vi "Draw Badges.vi"(8 "error in (no error)":errorcluster, 10 "picture in":picture, 11 "FSM in":refnum<class "FSM.Node.lvclass">) -> (0 "error out":errorcluster, 2 "picture out":picture, 3 "FSM out":refnum<class "FSM.Node.lvclass">)   [LabVIEW 2015, in "FSM.Node.lvclass"]
uses:
  FSM.Node.lvclass
  FSM.Node.lvclass/FSM.Node.ctl
  <vilib>/picture/picture.llb/Draw True-Color Pixmap.vi
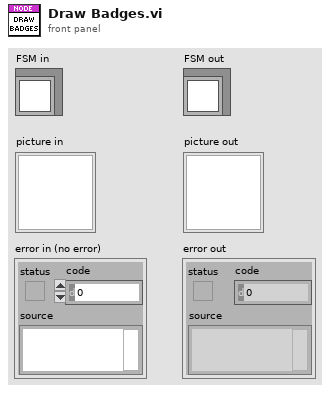
[diagram p1: front panel]
types:
  T1 = typedef "FSM.Node.lvclass/Badge.ctl" = enum16{"Audio", "Visual"}
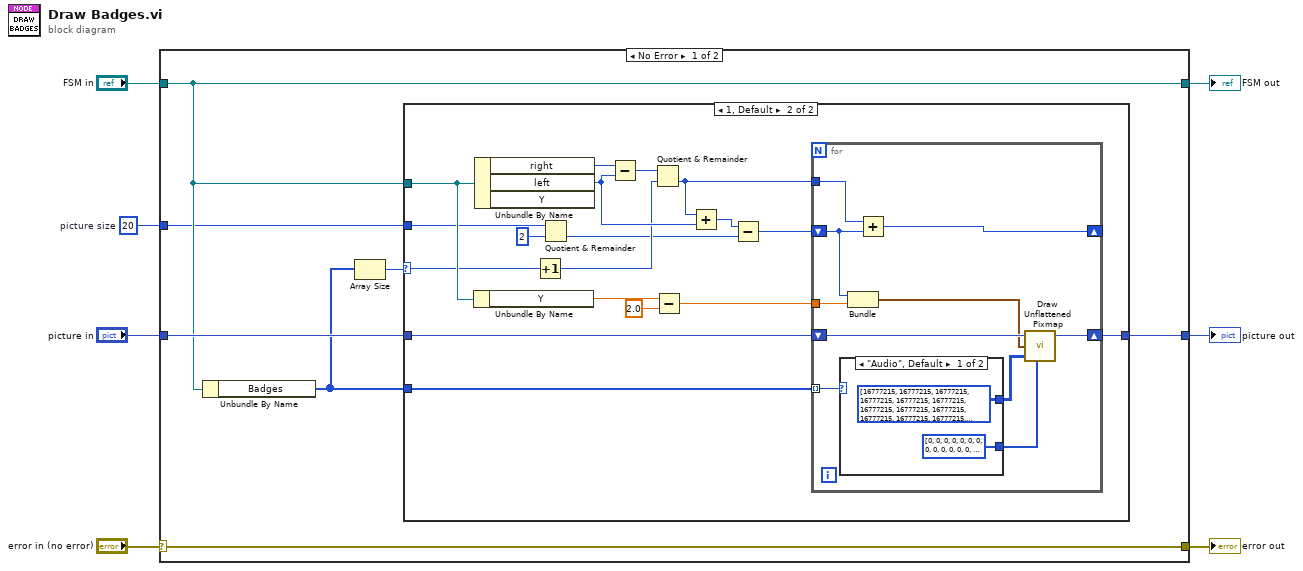
[diagram p0: block diagram]
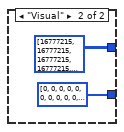
[diagram p3: hidden frame]
diagram:
  w1 = 20  # picture size
  n1 = case shown="No Error" "error in (no error)" {
    selector: "error in (no error)" -> [w14 w50]
    tunnel: [w14 w50] -> w6
    tunnel: [w11 w49] -> w4
    tunnel: "FSM in" -> [w11 w49]
    tunnel: "picture in" -> [w13 w48]
    tunnel: [w12 w48] -> w2
    tunnel: w1 -> [w9 _]
    frame No Error {
      n2 = Unbundle By Name(w11) -> ("Badges"=w8:T1[])
      n3 = Array Size(array=w8) -> (size(s)=w10:i32)
      n4 = case shown="1, Default" w10 {
        selector: w10 -> [_ w24]
        tunnel: w13 -> [w15 w31]
        tunnel: [w15 w30] -> w12
        tunnel: w11 -> [_ w27]
        tunnel: w9 -> [_ w23]
        tunnel: w8 -> [_ w20]
        frame 0 {
        }
        frame 1, Default {
          n5 = Unbundle By Name(w27) -> ("Y"=w26:dbl)
          n6 = Unbundle By Name(w27) -> ("right"=w33:i16, "left"=w29:i16)  [unwired: 1 out]
          n7 = Increment(x=w24) -> (x+1=w25:i32)
          n8 = Quotient & Remainder(x=w23, y=2) -> (floor(x/y)=w21:i32)  [unwired: 1 out]
          n9 = Subtract(x=w33, y=w29) -> (x-y=w32:i16)
          n10 = Quotient & Remainder(x=w32, y=w25) -> (floor(x/y)=w16:i32)  [unwired: 1 out]
          n11 = Subtract(x=w26, y=2.0) -> (x-y=w18:dbl)
          n12 = Add(x=w16, y=w29) -> (x+y=w17:i32)
          n13 = Subtract(x=w17, y=w21) -> (x-y=w19:i32)
          n14 = for {
            shift-right: [w42] -> w30
            shift-left: w31 -> [w43]
            tunnel: w20 -> [w34] mode=indexing
            tunnel: w18 -> [w39]
            tunnel: w16 -> [w37]
            shift-right: [w35] -> _
            shift-left: w19 -> [w36]
            n15 = case shown="\"Audio\", Default" w34 {
              tunnel: [u32[][] [[16777215, 16777215, 16777215, 16777215, 16777215, 16777215, 16777215, 16777215, 16777215, 16777215, 16777215, 16777215, 16777215, 16777215, 16777215, 16777215, 16777215, 16777215, 16777215, 16777215], [16777215, 16777215, 16777215, 16777215, 16777215, 16777215, 16777215, 16777215, 16777215, 16777215, 16777215, 16777215, 16777215, 16777215, 16777215, 16777215, 16777215, 16777215, 16777215, 16777215], [16777215, 16777215, 16777215, 16777215, 16777215, 16777215, 16777215, 16777215, 16777215, 16777215, 16777215, 16777215, 16777215, 16777215, 16777215, 16777215, 16777215, 16777215, 16777215, 16777215], [16777215, 16777215, 16777215, 16777215, 16777215, 16777215, 16777215, 16777215, 16777215, 16777215, 16777215, 16777215, 16777215, 16777215, 16777215, 16777215, 16777215, 16777215, 16777215, 16777215], [16777215, 16777215, 16777215, 5994709, 5994709, 5994709, 5994709, 5994709, 5863381, 5797332, 10464994, 14804723, 8228815, 12634601, 15922427, 16382718, 16514046, 16777215, 16777215, 16777215], [16777215, 16777215, 16777215, 4746200, 4746200, 4746200, 4746200, 4746200, 4811992, 4680665, 2772939, 4678084, 7439820, 14673139, 16054012, 16382717, 16514046, 16777215, 16777215, 16777215], [16777215, 16777215, 16777215, 1653428, 1653428, 1653428, 1653428, 1653428, 1653428, 1653684, 601519, 3232, 861346, 8229582, 16054012, 16711423, 16448254, 16777215, 16777215, 16777215], [16777215, 16777215, 16777215, 1192870, 1192870, 1192870, 1192870, 1192870, 929957, 1981867, 9280981, 4679099, 4502, 1425, 8491471, 16777215, 16777215, 16777215, 16777215, 16777215], [16777215, 16777215, 16777215, 1192866, 1192866, 1192866, 1192866, 1192866, 929952, 1653157, 9017810, 11911651, 9149652, 5782, 467610, 12897513, 16579839, 16777215, 16777215, 16777215], [16777215, 16777215, 16777215, 7319, 7320, 73112, 1192610, 1324451, 1258659, 798368, 535199, 8360655, 16777215, 11056862, 8599, 7638475, 15067894, 16777215, 16777215, 16777215], [16777215, 16777215, 16777215, 9609942, 9544149, 9084115, 1391267, 1062305, 1522339, 1522596, 8343, 5270459, 16579583, 16777215, 10005468, 3432123, 6061769, 16777215, 16777215, 16777215], [16777215, 16777215, 16777215, 16514046, 16185340, 16645375, 8492753, 538274, 998563, 1458597, 1064099, 801186, 10333915, 16777215, 14409973, 4614597, 3102654, 16777215, 16777215, 16777215], [16777215, 16777215, 16777215, 14936054, 14409970, 15133430, 12765932, 6455244, 343472, 671921, 1328819, 11944, 6521292, 12371434, 10859490, 10727905, 10727905, 16777215, 16777215, 16777215], [16777215, 16777215, 16777215, 14936054, 14475506, 14936053, 11451365, 10135518, 5798350, 608195, 805573, 13245, 10598888, 16777215, 16382461, 16645374, 16645374, 16777215, 16777215, 16777215], [16777215, 16777215, 16777215, 14936054, 14541555, 15527928, 11845863, 9413084, 8885715, 2777815, 1070811, 807384, 4553186, 15396859, 16776957, 16053755, 16053755, 16777215, 16777215, 16777215], [16777215, 16777215, 16777215, 15922427, 14804469, 10136288, 7835351, 6125258, 4152766, 2185940, 1924315, 2318298, 16851, 11913200, 16777214, 16053755, 16053755, 16777215, 16777215, 16777215], [16777215, 16777215, 16777215, 13883631, 10201050, 4743097, 3427498, 1983148, 1396684, 1726162, 1922510, 1856974, 1396940, 3368659, 15922684, 16447996, 15987963, 16777215, 16777215, 16777215], [16777215, 16777215, 16777215, 8491983, 6058425, 2637975, 2377636, 1858254, 1534962, 2778330, 3236046, 3105233, 2908112, 2776527, 11583466, 16645373, 16645373, 16777215, 16777215, 16777215], [16777215, 16777215, 16777215, 9215184, 5205946, 871351, 1993696, 1602041, 2189800, 10597090, 12897000, 12108775, 12174567, 11516900, 11517671, 16448253, 16711166, 16777215, 16777215, 16777215], [16777215, 16777215, 16777215, 12239585, 9808091, 2845659, 1730281, 4421857, 11845605, 16644342, 16381688, 16184567, 16184567, 16184567, 16184568, 16053755, 16053755, 16777215, 16777215, 16777215]] ("24-bit pixmap") u32[][] [[16777215, 16777215, 16777215, 16777215, 16777215, 16777215, 16777215, 16777215, 16777215, 16777215, 16777215, 16777215, 16777215, 16777215, 16777215, 16777215, 16777215, 16777215, 16777215, 16777215], [16777215, 16777215, 16777215, 16777215, 16777215, 16777215, 16777215, 16777215, 16777215, 16777215, 16777215, 16777215, 16777215, 16777215, 16777215, 16777215, 16777215, 16777215, 16777215, 16777215], [16777215, 16777215, 16777215, 16777215, 16777215, 16777215, 16777215, 16777215, 16777215, 16777215, 16777215, 16777215, 16777215, 16777215, 16777215, 16777215, 16777215, 16777215, 16777215, 16777215], [16777215, 16777215, 16777215, 16777215, 16777215, 16777215, 16777215, 16777215, 16777215, 16777215, 16777215, 16777215, 16777215, 16777215, 16777215, 16777215, 16777215, 16777215, 16777215, 16777215], [16777215, 16777215, 16777215, 16579059, 16117212, 15853272, 15852758, 15123848, 14858328, 14858055, 14857795, 14792277, 14992264, 15919065, 15787734, 16116440, 16447215, 16777215, 16777215, 16777215], [16777215, 16777215, 16777215, 16711422, 16315629, 15190938, 15055174, 15914307, 16311883, 16378705, 16443732, 16112968, 15516218, 14790467, 15190680, 16249322, 16579579, 16777215, 16777215, 16777215], [16777215, 16777215, 16777215, 16579322, 15719872, 14856244, 16245061, 16776291, 16776574, 16776612, 16776890, 16710288, 16445278, 15979070, 14855985, 15719354, 16447478, 16777215, 16777215, 16777215], [16777215, 16777215, 16777215, 15917516, 15122299, 15449901, 16642913, 16776876, 16777199, 16777215, 16777215, 16777209, 16710830, 16511073, 15582766, 15122804, 15719873, 16777215, 16777215, 16777215], [16777215, 16777215, 16777215, 15917517, 15188349, 15449899, 16511344, 16776931, 16777215, 16777215, 16777215, 16777215, 16777204, 16643466, 15649582, 15254386, 15719357, 16777215, 16777215, 16777215], [16777215, 16777215, 16777215, 16380911, 15455145, 15054382, 16246105, 16776136, 16777215, 16777215, 16777215, 16777215, 16777205, 16576902, 15384363, 15322262, 16116449, 16777215, 16777215, 16777215], [16777215, 16777215, 16777215, 16711679, 16381683, 14989919, 15715127, 16511344, 16776385, 16777201, 16777210, 16777198, 16776107, 16112712, 15055954, 16051170, 16381687, 16777215, 16777215, 16777215], [16777215, 16777215, 16777215, 16711423, 16711679, 15588029, 14922814, 16311115, 16709987, 16710786, 16710800, 16776064, 16576344, 15254072, 15389612, 16447737, 16381683, 16777215, 16777215, 16777215], [16777215, 16777215, 16777215, 16513782, 16513783, 15985637, 15255431, 15978044, 16710748, 16777046, 16777044, 16645205, 16243258, 15255417, 15721171, 16315115, 16315115, 16777215, 16777215, 16777215], [16777215, 16777215, 16777215, 16775664, 16775664, 16777215, 15919585, 15059536, 16777033, 16777037, 16183611, 16314422, 15190853, 16115413, 16775926, 16774117, 16774117, 16777215, 16777215, 16777215], [16777215, 16777215, 16777215, 13554904, 13554904, 13686490, 13687014, 10003090, 7960635, 10526313, 15854516, 14079385, 10332568, 13094873, 13423574, 13291988, 13291988, 16777215, 16777215, 16777215], [16777215, 16777215, 16777215, 11123138, 11123138, 11057345, 11781324, 10267324, 5660535, 7634322, 14278901, 12437212, 9741494, 10926016, 10531258, 10597051, 10597051, 16777215, 16777215, 16777215], [16777215, 16777215, 16777215, 12306379, 12306379, 12306379, 12898773, 10464175, 7304825, 9804442, 13818073, 11910075, 10397096, 12305865, 11976643, 11976643, 11976643, 16777215, 16777215, 16777215], [16777215, 16777215, 16777215, 11912651, 11912651, 11912651, 12439252, 10793655, 6251363, 8159360, 14212573, 10660008, 10595505, 12240845, 11911623, 11911623, 11911623, 16777215, 16777215, 16777215], [16777215, 16777215, 16777215, 14542827, 14542827, 14542827, 15661051, 11977929, 2041898, 6383720, 9608349, 4608337, 13292758, 15923450, 15068398, 15068398, 15068398, 16777215, 16777215, 16777215], [16777215, 16777215, 16777215, 16383229, 16383229, 16383229, 16777215, 14278367, 9805731, 9938346, 10727604, 11778489, 14869988, 16777215, 16777215, 16777215, 16777215, 16777215, 16777215, 16777215]] ("24-bit pixmap")] -> w41
              tunnel: [u8[] [0, 0, 0, 0, 0, 0, 0, 0, 0, 0, 0, 0, 0, 0, 0, 0, 0, 96, 0, 0, 0, 112, 0, 0, 0, 124, 0, 0, 0, 126, 0, 0, 0, 78, 0, 0, 0, 67, 0, 0, 0, 67, 0, 0, 0, 65, 0, 0, 0, 64, 0, 0, 0, 64, 0, 0, 0, 64, 0, 0, 7, 192, 0, 0, 15, 192, 0, 0, 31, 192, 0, 0, 15, 128, 0, 0, 7, 0, 0, 0] ("mask") u8[] [0, 0, 0, 0, 0, 0, 0, 0, 0, 0, 0, 0, 0, 0, 0, 0, 1, 248, 0, 0, 3, 254, 0, 0, 7, 254, 0, 0, 15, 255, 0, 0, 15, 255, 0, 0, 7, 255, 0, 0, 7, 254, 0, 0, 3, 252, 0, 0, 3, 252, 0, 0, 1, 248, 0, 0, 1, 248, 0, 0, 1, 248, 0, 0, 1, 248, 0, 0, 1, 248, 0, 0, 0, 240, 0, 0, 0, 96, 0, 0] ("mask")] -> w40
              frame "Audio", Default {
              }
              frame "Visual" {
              }
            }
            n16 = Bundle(w36, w39) -> (w38:cluster{i32, dbl})  [unwired: 1 in]
            n17 = Add(x=w37, y=w36) -> (x+y=w35:i32)
            n18 = call-poly <vilib>:"Draw Unflattened Pixmap.vi"("picture"=w43, "top left point(0, 0)"=w38, "data (RGB format)"=w41, "mask"=w40) -> ("new picture"=w42:picture)  [unwired: 5 in]
          }
        }
      }
    }
    frame Error {
    }
  }
  "error out" <- w6
  "FSM out" <- w4
  "picture out" <- w2
